vi "lissaaa.vi"() -> ()   [LabVIEW 2011]
panel:
  out "XY Graph":cluster{"Y":dbl[], "Y":dbl[]}[](graph)
  in  "phase 1":dbl
  in  "fre 1":dbl
  in  "Amp 1":dbl
  in  "phase":dbl
  in  "frequency":dbl
  in  "Amp":dbl
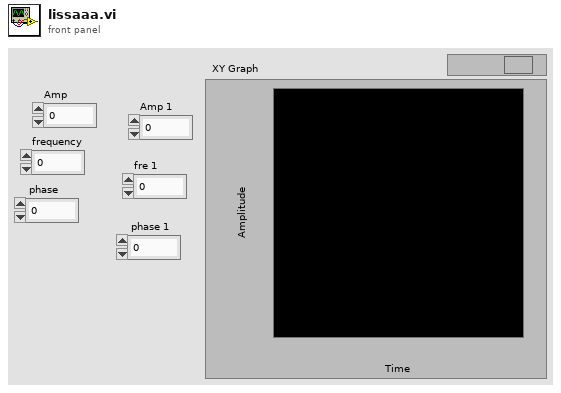
[diagram p1: front panel]
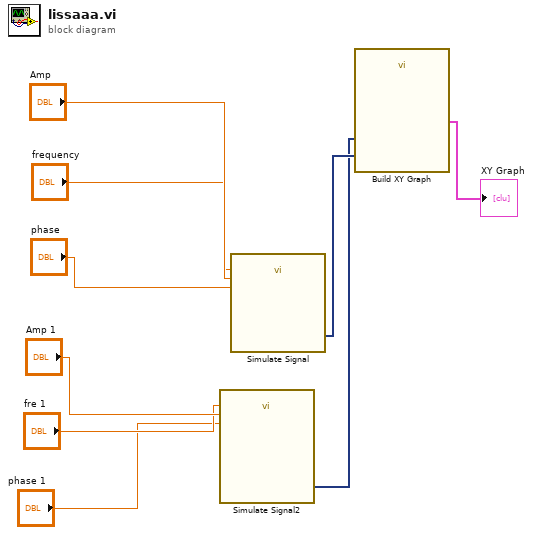
[diagram p0: block diagram]
diagram:
  n1 = call "Simulate Signal2"("Frequency"="fre 1", "Amplitude"="Amp 1", "Phase"="phase 1") -> ("Sine"=w1:dynamicdata)  [unwired: 11 in, 1 out]
  n2 = call "Simulate Signal"("Frequency"="frequency", "Amplitude"="Amp", "Phase"="phase") -> ("Sine"=w5:dynamicdata)  [unwired: 11 in, 1 out]
  n3 = call "Build XY Graph"("Y Input"=w1, "X Input"=w5) -> ("XY Graph"=→"XY Graph":cluster{"Y":dbl[], "Y":dbl[]}[])  [unwired: 3 in, 6 out]
